vi "generate_input_surface.vi"(10 "y":dbl) -> (0 "z matrix":dbl[][](array[numeric]), 1 "Y Vector":dbl[](array[numeric]), 2 "X Vector":dbl[](array[numeric]))   [LabVIEW 2020, in "3DPC_SurfacePlot.xctl"]
uses:
  <vilib>/Native 3D Graph/xcontrol/3DPC_SurfacePlot.xctl
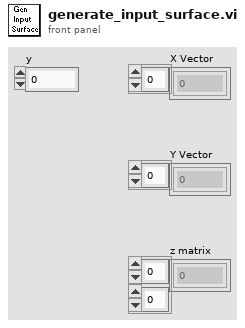
[diagram p1: front panel]
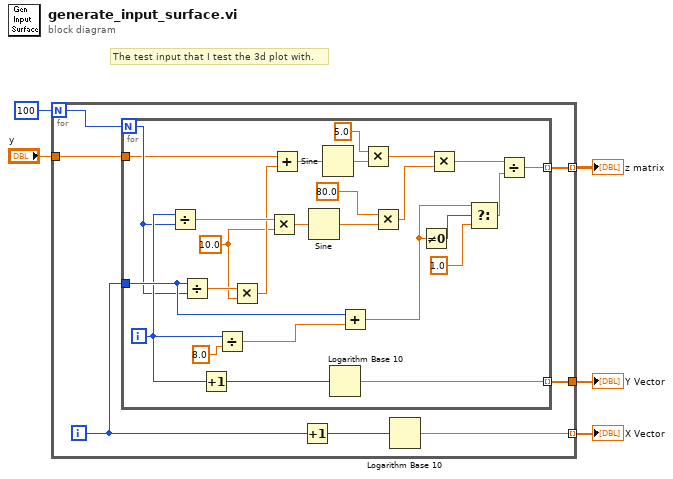
[diagram p0: block diagram]
diagram:
  # "The test input that I test the 3d plot with."
  n1 = for {
    N: 100 -> [w7]
    tunnel: [w9] -> w5
    tunnel: [w10] -> w4 mode=indexing
    tunnel: [w8] -> w2 mode=indexing
    tunnel: "y" -> [w6]
    i -> [w12]
    n2 = for {
      N: w7 -> [w17]
      tunnel: w12 -> [w26]
      tunnel: [w16] -> w10 mode=indexing
      tunnel: [w15] -> w9 mode=indexing
      tunnel: w6 -> [w14]
      i -> [w20]
      w13 = 10.0 ("x")
      n3 = Divide(x=w20, y=w17) -> (x/y=w37:dbl)
      n4 = Divide(x=w26, y=w17) -> (x/y=w35:dbl)
      n5 = Increment(x=w20) -> (x+1=w23:i32)
      n6 = Divide(x=w20, y=8.0) -> (x/y=w18:dbl)
      n7 = Multiply(x=w35, y=w13) -> (x*y=w34:dbl)
      n8 = Multiply(x=w37, y=w13) -> (x*y=w36:dbl)
      n9 = Add(x=w14, y=w34) -> (x+y=w28:dbl)
      n10 = Sine(x=w36) -> (sin(x)=w31:dbl)
      n11 = Sine(x=w28) -> (sin(x)=w38:dbl)
      n12 = Logarithm Base 10(1:w23) -> (0:w15:dbl)
      n13 = Add(x=w26, y=w18) -> (x+y=w21:dbl)
      n14 = Multiply(x=5.0, y=w38) -> (x*y=w33:dbl)
      n15 = Multiply(x=80.0, y=w31) -> (x*y=w30:dbl)
      n16 = Not Equal To 0?(x=w21) -> (x != 0?=w25:bool)
      n17 = Multiply(x=w33, y=w30) -> (x*y=w27:dbl)
      n18 = Select(t=w21, s=w25, f=1.0) -> (s? t:f=w22:dbl)
      n19 = Divide(x=w27, y=w22) -> (x/y=w16:dbl)
    }
    n20 = Increment(x=w12) -> (x+1=w11:i32)
    n21 = Logarithm Base 10(1:w11) -> (0:w8:dbl)
  }
  "z matrix" <- w4
  "Y Vector" <- w5
  "X Vector" <- w2
